vi "env_read_data.vi"(8 "error in":errorcluster, 9 "Input parameters":T1, 10 "State":T2, 11 "Stop signal":T4) -> (0 "error out":errorcluster, 2 "Plot data out":T3, 3 "Env data out":T5)   [LabVIEW 2016]
doc: "Reads out the environmental sensors."
uses:
  <extravilib>/ChannelInstances/Tag-t'Env_data.ctl'/))Channel.ctl
  data_env.ctl
  <extravilib>/ChannelInstances/Tag-bool/))Channel.ctl
  <extravilib>/ChannelInstances/Tag-a[.](c(a[.](stamp),a[.](dbl)))/))Channel.ctl
  <extravilib>/ChannelInstances/Tag-str/))Channel.ctl
  <extravilib>/ChannelInstances/Tag-t'Input_parameters.ctl'/))Channel.ctl
  input_params.ctl
  <extravilib>/ChannelInstances/Tag-t'Input_parameters.ctl'/Read With Abort.vi
  <extravilib>/ChannelInstances/Tag-str/Read With Abort.vi
  <extravilib>/ChannelInstances/Tag-bool/Read With Abort.vi
  <extravilib>/ChannelInstances/Tag-t'Env_data.ctl'/Write With Abort.vi
  <extravilib>/ChannelInstances/Tag-a[.](c(a[.](stamp),a[.](dbl)))/Write With Abort.vi
  <extravilib>/ChannelInstances/Tag-t'Input_parameters.ctl'/Endpoint.vi
  <extravilib>/ChannelInstances/Tag-str/Endpoint.vi
  <extravilib>/ChannelInstances/Tag-bool/Endpoint.vi
  <extravilib>/ChannelInstances/Tag-t'Env_data.ctl'/Endpoint.vi
  <extravilib>/ChannelInstances/Tag-a[.](c(a[.](stamp),a[.](dbl)))/Endpoint.vi
  <instrlib>/iowkit.dll
  <extravilib>/ChannelInstances/Tag-bool.lvlib
  <extravilib>/ChannelInstances/Tag-t'Env_data.ctl'.lvlib
  <extravilib>/ChannelInstances/Tag-a[.](c(a[.](stamp),a[.](dbl))).lvlib
  <extravilib>/ChannelInstances/Tag-str.lvlib
  <extravilib>/ChannelInstances/Tag-t'Input_parameters.ctl'.lvlib
panel:
  out "Probecard temperature":dbl
  out "Probecard humidity":dbl
  out "Switchboard Handle":u32
  out "Ask switchboard?":bool
  out "External humidity":sgl
  out "External temperature":sgl
  out "Matrix temperature":dbl
  out "Matrix humidity":dbl
  in  "Sample period (s)":sgl=2.0
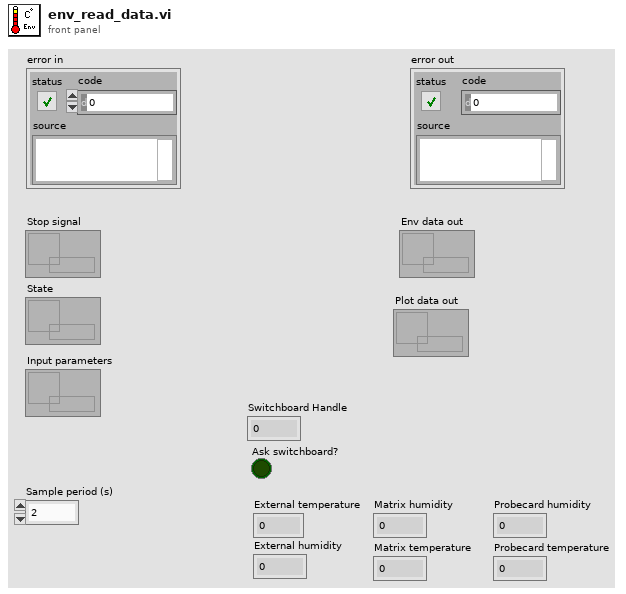
[diagram p1: front panel]
types:
  T1 = typedef "Tag-t'Input_parameters.ctl'.lvlib/))Channel.ctl" = refnum<queue>
  T2 = typedef "Tag-str.lvlib/))Channel.ctl" = refnum<queue>
  T3 = typedef "Tag-a[.](c(a[.](stamp),a[.](dbl))).lvlib/))Channel.ctl" = refnum<queue>
  T4 = typedef "Tag-bool.lvlib/))Channel.ctl" = refnum<queue>
  T5 = typedef "Tag-t'Env_data.ctl'.lvlib/))Channel.ctl" = refnum<queue>
  T6 = typedef "data_env.ctl" = cluster{"Temp. Sensirion":dbl, "Hum. Sensirion":dbl, "Temp. Switch Matrix":dbl, "Hum. Switch Matrix":dbl, "Temp. Probecard":dbl, "Hum. Probecard":dbl}
  T7 = typedef "input_params.ctl" = cluster{"Measurement type":enum16{"IV", "CV", "Debug", "Test_contact"}, "Sensor type":enum16{"HPK_6in_135", "HPK_8in_256", "IFX_8in_256", "Diode", "HPK_6in_256", "Full matrix"}, "Identifier":string, "Open after execution?":bool, "Plot after execution?":bool, "Display channel":i32, "Voltage Delay (s)":dbl, "Switch Delay (s)":dbl, "VISA resource name source":refnum<visa-resource-name>, "VISA resource name DMM":refnum<visa-resource-name>, "VISA resource name LCR":refnum<visa-resource-name>, "Compliance  Level (A)":dbl, "Voltage Limit (V)":dbl, "Data storage location":string, "Scan voltages":string, "Use source as DMM?":bool, "LCR signal frequenzy (Hz)":dbl, "DMM device":enum16{"Keithley2001", "Keithley2450", "Keithley2410", "Keithley6487"}, "Sampling number":i32, "Use env. sensors on":enum16{"Sensirion sht1x/7x", "Switch Matrix", "Probecard"}, "Switchboard Handle":u32, "Use Switchboard":bool, "LCR signal voltage (V)":dbl, "Repeat":i32, "Scan voltages IV":string, "Scan voltages CV":string, "Hex pad numbers?":bool, "Set measurement type":enum16{"IV", "CV", "Debug", "Test_contact", "IV+CV"}, "Custom pad scan":string, "IV voltage Delay (s)":dbl, "CV voltage Delay (s)":dbl, "Needle measurement?":bool, "Comments":string, "LCR signal frequenzy (kHz)":dbl, "Compliance  Level (uA)":dbl, "Open Correction Array":dbl[][], "Current set voltage":dbl, "Last set voltage":dbl, "Current channel":i32, "Last OpenCorrection index":i32, "Total curr/vltg every x steps":i32, "Current channel iteration":i32, "No CV corrections":bool, "Mapfile":string, "Corrfile":string, "IV voltage file":path, "CV voltage file":path, "IV Switch Delay (s)":dbl, "CV Switch Delay (s)":dbl, "Invert polarity":bool, "Set debug dirs":bool, "Is n on p":bool}
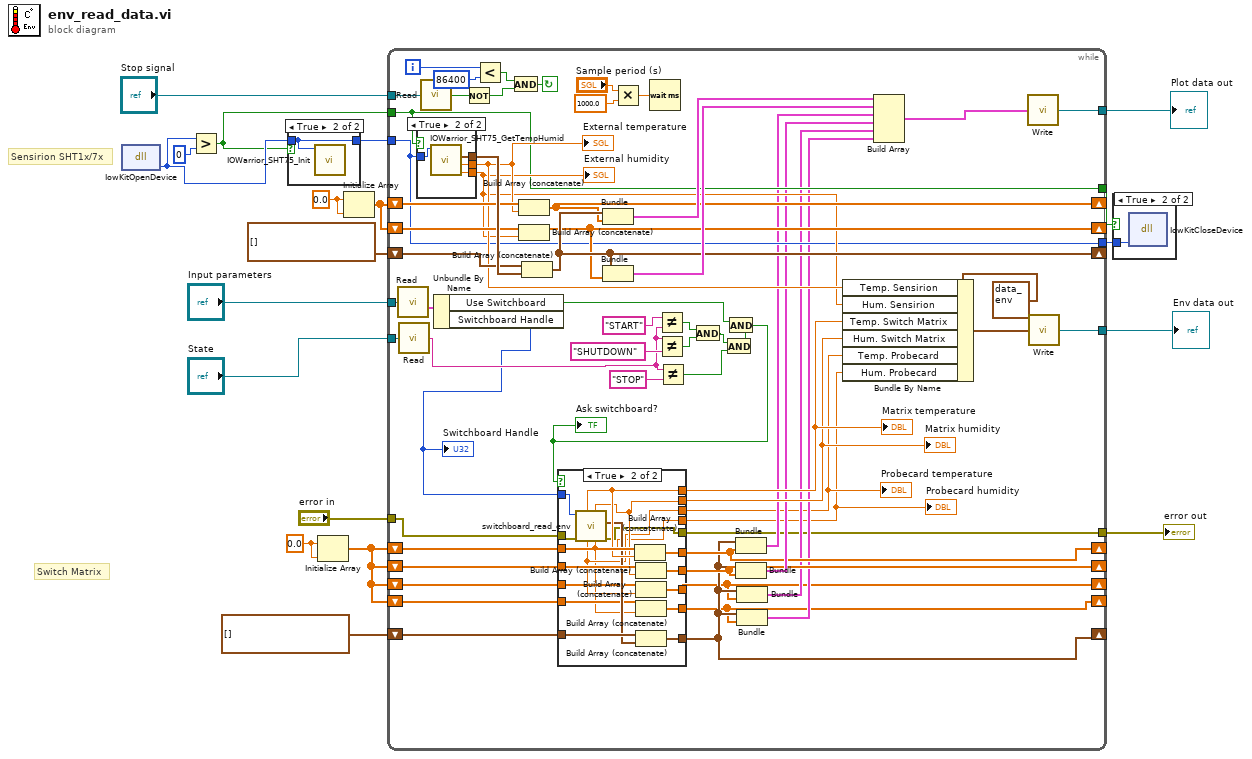
[diagram p0: block diagram]
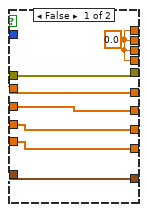
[diagram p4: hidden frame]
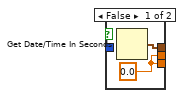
[diagram p5: hidden frame]
diagram:
  w6 = 0.0
  w13 = 0.0
  # "Switch Matrix"
  # "Sensirion SHT1x/7x"
  n1 = dll-call lib="C:/Program Files (x86)/National Instruments/LabVIEW 2016/instr.lib/iowkit.dll" fn="IowKitOpenDevice"() -> ("return type"=w10:i64)  [unwired: 3 in, 2 out]
  n2 = Greater?(x=w10, y=0) -> (0:w9:bool)
  n3 = case shown="True" w9 {
    tunnel: w10 -> [w19 w20]
    tunnel: [w19 w20] -> _
    frame False {
    }
    frame True {
      n4 = call <instrlib>:"IOWarrior_SHT75_Init.vi"("Dongle handle"=w20) -> ()  [unwired: 11 out]
    }
  }
  n5 = Initialize Array(w6, w6) -> (w3:dbl[])
  n6 = Initialize Array(w13, w13) -> (w12:dbl[])
  n7 = while {
    tunnel: w10 -> [w62]
    shift-right: [w72] -> _
    shift-left: w12 -> [w76]
    shift-right: [w71] -> _
    shift-left: w12 -> [w75]
    shift-right: [w73] -> _
    shift-left: timestamp[] [] -> [w74]
    tunnel: "Stop signal" -> [w70]
    tunnel: [w66] -> w17
    tunnel: [w62] -> w14
    tunnel: [w61] -> w15
    tunnel: w9 -> [w57]
    tunnel: [w57] -> w8
    tunnel: "State" -> [w54]
    shift-right: [w39] -> _
    shift-left: w3 -> [w51]
    shift-right: [w41] -> _
    shift-left: w3 -> [w42]
    shift-right: [w29] -> _
    shift-left: timestamp[] [] -> [w40]
    tunnel: "Input parameters" -> [w35]
    shift-right: [w26] -> _
    shift-left: w3 -> [w31]
    shift-right: [w25] -> _
    shift-left: w3 -> [w30]
    tunnel: "error in" -> [w22]
    tunnel: [w21] -> w1
    i -> [w65]
    stop <- w80 continue-if-true
    n8 = call <extravilib>:"Read.vi"("channel"=w35) -> ("element"=w34:T7)  [unwired: 1 in, 1 out]
    n9 = call <extravilib>:"Read.vi"("channel"=w54) -> ("element"=w36:string)  [unwired: 1 in, 1 out]
    n10 = case shown="True" w57 {
      tunnel: [w109 w114] -> w77
      tunnel: [w110 w113] -> w64
      tunnel: [w110 w112] -> w63
      tunnel: w62 -> [_ w111]
      frame False {
        w110 = sgl 0.0 ("Temperature")
        n11 = Get Date/Time In Seconds() -> (seconds since 1Jan1904=w109:timestamp)
      }
      frame True {
        n12 = call <instrlib>:"IOWarrior_SHT75_GetTempHumid.vi"("Dongle handle"=w111) -> ("Humidity"=w112:sgl, "Temperature"=w113:sgl, "Time Stamp"=w114:timestamp)  [unwired: 7 out]
      }
    }
    "External temperature" <- w64
    "External humidity" <- w63
    n13 = call <extravilib>:"Read.vi"("channel"=w70) -> ("element"=w69:bool)  [unwired: 1 in, 1 out]
    n14 = Unbundle By Name(w34) -> ("Use Switchboard"=w33:bool, "Switchboard Handle"=w32:u32)
    "Switchboard Handle" <- w32
    n15 = Not(x=w69) -> (.not. x?=w83:bool)
    n16 = Less?(x=w65, y=86400) -> (x < y?=w82:bool)
    n17 = And(x=w82, y=w83) -> (x .and. y?=w80:bool)
    n18 = Build Array (concatenate)(w76, w64) -> (w72:dbl[])
    n19 = Build Array (concatenate)(w75, w63) -> (w71:dbl[])
    n20 = Build Array (concatenate)(w74, w77) -> (w73:timestamp[])
    n21 = Bundle(w73, w72) -> (w79:cluster{timestamp[], dbl[]})  [unwired: 1 out]
    n22 = Bundle(w73, w71) -> (w78:cluster{timestamp[], dbl[]})  [unwired: 1 out]
    n23 = Multiply(x="Sample period (s)", y=sgl 1000.0) -> (x*y=w60:sgl)
    n24 = Wait (ms)(milliseconds to wait=w60) -> ()  [unwired: 1 out]
    n25 = Not Equal?(x="START", y=w36) -> (x != y?=w55:bool)
    n26 = Not Equal?(x=w36, y="SHUTDOWN") -> (x != y?=w56:bool)
    n27 = Not Equal?(x=w36, y="STOP") -> (x != y?=w37:bool)
    n28 = And(x=w55, y=w56) -> (x .and. y?=w46:bool)
    n29 = And(x=w46, y=w37) -> (x .and. y?=w45:bool)
    n30 = And(x=w33, y=w45) -> (x .and. y?=w38:bool)
    "Ask switchboard?" <- w38
    n31 = case shown="True" w38 {
      tunnel: w32 -> [_ w108]
      tunnel: w51 -> [w88 w107]
      tunnel: [w85 w103] -> w50
      tunnel: [w85 w102] -> w49
      tunnel: w42 -> [w89 w106]
      tunnel: [w89 w100] -> w41
      tunnel: w40 -> [w90 w105]
      tunnel: [w90 w104] -> w29
      tunnel: [w88 w99] -> w39
      tunnel: w31 -> [w87 w95]
      tunnel: w30 -> [w86 w96]
      tunnel: [w87 w98] -> w26
      tunnel: [w86 w97] -> w25
      tunnel: [w85 w94] -> w24
      tunnel: [w85 w93] -> w23
      tunnel: w22 -> [w84 w92]
      tunnel: [w84 w91] -> w21
      frame False {
        w85 = 0.0 ("Matrix temperature")
      }
      frame True {
        n32 = call "switchboard_read_env.vi"("error in"=w92, "Handle"=w108) -> ("error out"=w91:errorcluster, "current time"=w101:timestamp, "Probecard humidity"=w93:dbl, "Matrix humidity"=w102:dbl, "Probecard temperature"=w94:dbl, "Matrix temperature"=w103:dbl)  [unwired: 3 in, 1 out]
        n33 = Build Array (concatenate)(w107, w103) -> (w99:dbl[])
        n34 = Build Array (concatenate)(w106, w102) -> (w100:dbl[])
        n35 = Build Array (concatenate)(w95, w94) -> (w98:dbl[])
        n36 = Build Array (concatenate)(w96, w93) -> (w97:dbl[])
        n37 = Build Array (concatenate)(w105, w101) -> (w104:timestamp[])
      }
    }
    "Matrix humidity" <- w49
    "Matrix temperature" <- w50
    "Probecard humidity" <- w23
    "Probecard temperature" <- w24
    n38 = Bundle(w29, w39) -> (w48:cluster{timestamp[], dbl[]})  [unwired: 1 out]
    n39 = Bundle(w29, w41) -> (w43:cluster{timestamp[], dbl[]})  [unwired: 1 out]
    n40 = Bundle(w29, w26) -> (w28:cluster{timestamp[], dbl[]})  [unwired: 1 out]
    n41 = Bundle(w29, w25) -> (w27:cluster{timestamp[], dbl[]})  [unwired: 1 out]
    n42 = Bundle By Name(cluster=T6 {"Temp. Sensirion"=0.01, "Hum. Sensirion"=0.01, "Temp. Switch Matrix"=0.01, "Hum. Switch Matrix"=0.01, "Temp. Probecard"=0.01, "Hum. Probecard"=0.01} ("Cluster"), "Temp. Sensirion"=w64, "Hum. Sensirion"=w63, "Temp. Switch Matrix"=w50, "Hum. Switch Matrix"=w49, "Temp. Probecard"=w24, "Hum. Probecard"=w23) -> (w68:T6)
    n43 = Build Array(w79, w78, w48, w43, w28, w27) -> (w44:cluster{timestamp[], dbl[]}[])
    n44 = call <extravilib>:"Write.vi"("element"=w44) -> ("channel"=w61:T3)  [unwired: 1 out]
    n45 = call <extravilib>:"Write.vi"("element"=w68) -> ("channel"=w66:T5)  [unwired: 1 out]
  }
  "Env data out" <- w17
  "Plot data out" <- w15
  "error out" <- w1
  n46 = case shown="True" w8 {
    tunnel: w14 -> [_ w115]
    frame False {
    }
    frame True {
      n47 = dll-call lib="C:/Program Files (x86)/National Instruments/LabVIEW 2016/instr.lib/iowkit.dll" fn="IowKitCloseDevice"("devHandle"=w115) -> ()  [unwired: 3 in, 4 out]
    }
  }
